vi "client-test2.vi"() -> ()   [LabVIEW 2016]
doc: "client test for TCP server in Main."
uses:
  <vilib>/NI/STM/TCP/TCP Read Options.ctl
  <vilib>/NI/STM/TCP/Read Meta Data (TCP Ref).vi
  <vilib>/NI/STM/TCP/Get Connection Reference (TCP).vi
  <vilib>/NI/STM/TCP/Read Meta Data (TCP Clst).vi
  <vilib>/NI/STM/TCP/Read Message (TCP).vi
  <vilib>/NI/STM/NI STM.lvlib
  <vilib>/NI/STM/TCP/Write Message (TCP).vi
panel:
  out "data string":string
  out "error  out":errorcluster
  in  "stop":bool
  in  "Target IP Address":string="localhost"
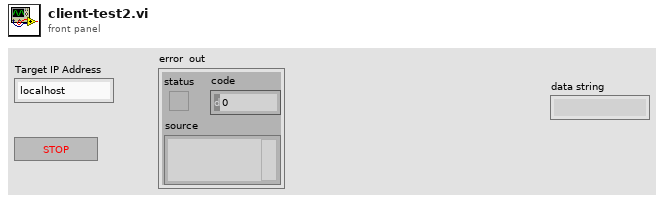
[diagram p1: front panel]
types:
  T1 = typedef "NI STM.lvlib/TCP Connection Info.ctl" = cluster{"connection ID":refnum<k5>, "meta data":T2[]}
  T2 = typedef "NI STM.lvlib/MetaDataElement.ctl" = string
  T3 = typedef "NI STM.lvlib/TCP Read Options.ctl" = cluster{"ignore timeout error":bool, "timeout ms (1000)":i32}
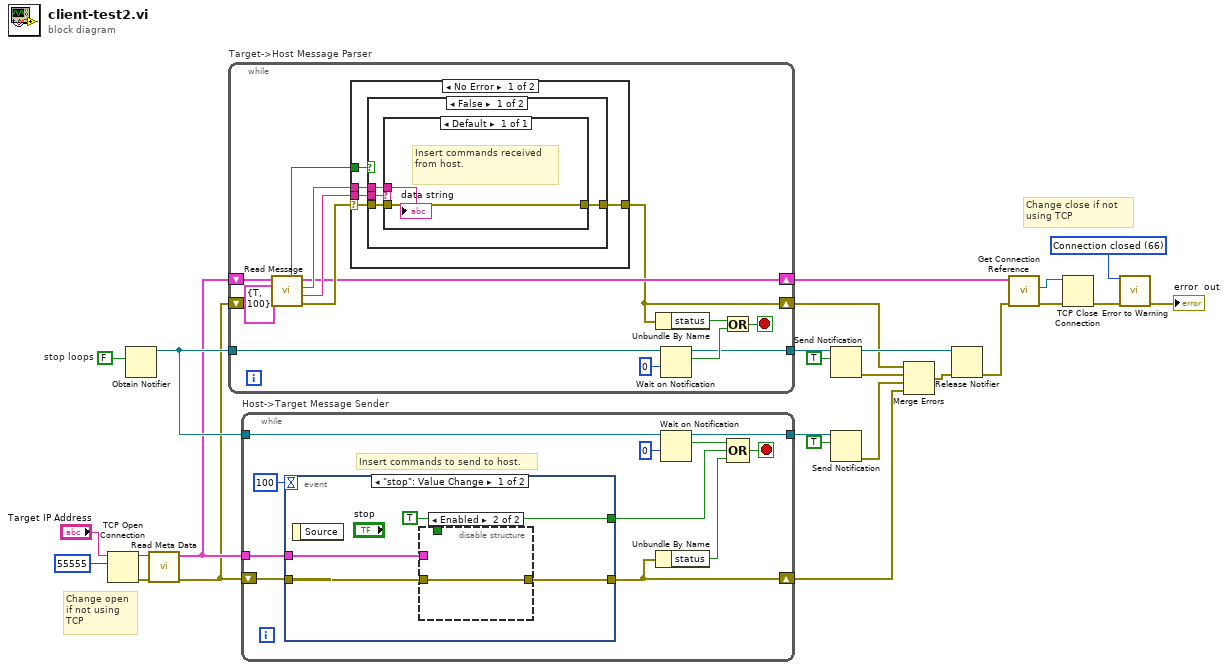
[diagram p0: block diagram]
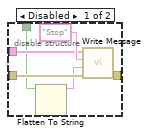
[diagram p2: hidden frame]
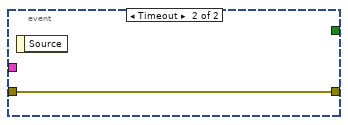
[diagram p3: hidden frame]
diagram:
  w11 = FALSE  # stop loops
  w23 = 66 items=["No Error", "Argument Error", "Memory Full", "Out of Zone", "End of File", "File Already Open", "Generic File IO Error", "File Not Found", "File Permission Error", "Disk Full", "Duplicate Path", "Too Many Files Open", "Not Enabled", "Resource File Not Found", "Cannot Add Resource", "Resource Not Found", "Image Not Found", "Image Memory Error", "Pen Does Not Exist", "Config Bad Type", "Config Token Not Found", "Config Parse Error", "Config Memory Error", "Bad External Code Format", "Bad External Code Offset", "External Code Not Present", "Null Window", "Destroy Window Mixup", "Null Menu", "Print Aborted", "Bad Print Record", "Print Driver Error", "Windows Error During Print", "Memory Error During Print", "Print Dialog Error", "Generic Print Error", "Invalid Device Refnum", "Device Not Found", "Device Parameter Error", "Device Unit Error", "Can't Open Device", "Device Call Aborted", "Generic Error", "Cancelled By User", "Object ID Too Low", "Object ID Too High", "Object Not In Heap", "Unknown Heap", "Bad DefProc ID", "DefProc Not In Table", "Message Out Of Range", "Null Method", "Unknown Message", "Manager Call Not Supported", "Bad address", "Connection In progress", "Connection timed out", "Connection is already in progress", "Network attribute not supported", "Network error", "Address in use", "System out of memory", "Connection aborted", "Connection refused", "Connection is not connected", "Connection is already connected", "Connection closed", "Initialize error (interapplication manager)", "Bad occurrence", "Wait on unbound occurrence handler", "Occurrence queue overflow", "Bad path", "Semaphore not signaled", "Unrecognized type (interapplication manager)"] ("1st Error to Convert")
  # "Change close if not using TCP"
  # "Change open if not using TCP"
  n1 = TCP Open Connection(address="Target IP Address", remote port or service name=u16 55555 ("remote port")) -> (connection ID=w7:refnum<k5>, error out=w6:errorcluster)  [unwired: 1 in, 2 out]
  n2 = Obtain Notifier(notification data type=w11) -> (notifier out=w14:refnum<notifier>)  [unwired: 3 in, 2 out]
  n3 = call-poly <vilib>:"Read Meta Data.vi"("error in"=w6, "connection ID"=w7) -> ("error out"=w8:errorcluster, "connection info out"=w9:T1)  [unwired: 1 in, 7 out]
  n4 = while "Target->Host Message Parser" {
    shift-right: [w27] -> w3
    shift-left: w8 -> [w39]
    tunnel: w14 -> [w33]
    tunnel: [w29] -> w12
    shift-right: [w34] -> w10
    shift-left: w9 -> [w40]
    stop <- w30 stop-if-true
    n5 = call-poly <vilib>:"Read Message.vi"("options"=T3 {"ignore timeout error"=TRUE, "timeout ms (1000)"=100}, "error in"=w39, "connection info in"=w40) -> ("error out"=w35:errorcluster, "name"=w38:T2, "data string"=w37:string, "connection info out"=w34:T1, "timed out?"=w36:bool)  [unwired: 2 in, 2 out]
    n6 = case shown="No Error" w35 {
      selector: w35 -> [w42 w53]
      tunnel: w38 -> [w45 _]
      tunnel: w37 -> [w44 _]
      tunnel: w36 -> [w43 _]
      tunnel: [w41 w53] -> w27
      frame No Error {
        n7 = case shown="False" w43 {
          tunnel: w45 -> [w46 _]
          tunnel: w44 -> [w49 _]
          tunnel: w42 -> [w48 w52]
          tunnel: [w47 w52] -> w41
          frame False {
            n8 = case shown="Default" w46 {
              tunnel: w49 -> [w50]
              tunnel: w48 -> [w51]
              tunnel: [w51] -> w47
              frame Default {
                # "Insert commands received from host."
                "data string" <- w50
              }
            }
          }
          frame True {
          }
        }
      }
      frame Error {
      }
    }
    n9 = Unbundle By Name(w27) -> ("status"=w28:bool)
    n10 = Wait on Notification(notifier=w33, timeout in ms (-1)=0) -> (notifier out=w29:refnum<notifier>, notification=w31:bool)  [unwired: 2 in, 2 out]
    n11 = Or(x=w28, y=w31) -> (x .or. y?=w30:bool)
  }
  n12 = while "Host->Target Message Sender" {
    shift-right: [w56] -> w17
    shift-left: w8 -> [w64]
    tunnel: w9 -> [w63]
    tunnel: w14 -> [w60]
    tunnel: [w57] -> w15
    stop <- w58 stop-if-true
    # "Insert commands to send to host."
    n13 = event shown="[0] \"stop\": Value Change" {
      selector: _ -> [_ _]
      dyn-events: _ -> [_ _]
      timeout: 100 -> [_ _]
      tunnel: w63 -> [w68 _]
      tunnel: w64 -> [w67 w76]
      tunnel: [w66 _] -> w55
      tunnel: [w65 w76] -> w56
      event "stop": Value Change {
        w66 = TRUE ("stop")
        n14 = event-data() -> ()  [unwired: 2 out]
        n15 = disable-structure shown="Enabled" {
          disable-tunnel: w68 -> [w73 _]
          disable-tunnel: w67 -> [w72 w75]
          disable-tunnel: w66 -> [w70 _]
          disable-tunnel: [w69 w75] -> w65
          frame Disabled {
            n16 = Flatten To String(anything=w70) -> (data string=w71:string)  [unwired: 2 in, 3 out]
            n17 = call-poly <vilib>:"Write Message.vi"("error in"=w72, "data"=w71, "name"="Stop" ("Name"), "connection info in"=w73) -> ("error out"=w69:errorcluster)  [unwired: 1 in, 6 out]
          }
          frame Enabled {
          }
        }
      }
      event Timeout {
        n18 = event-data() -> ()  [unwired: 2 out]
      }
    }
    n19 = Unbundle By Name(w56) -> ("status"=w54:bool)
    n20 = Wait on Notification(notifier=w60, timeout in ms (-1)=0) -> (notifier out=w57:refnum<notifier>, notification=w62:bool)  [unwired: 2 in, 2 out]
    n21 = Compound Arithmetic op=OR(w62, w55, w54) -> (w58:bool)
  }
  n22 = Send Notification(notification=TRUE, notifier=w12) -> (notifier out=w20:refnum<notifier>, error out=w19:errorcluster)  [unwired: 1 in]
  n23 = Send Notification(notification=TRUE, notifier=w15) -> (error out=w18:errorcluster)  [unwired: 1 in, 1 out]
  n24 = Merge Errors(w3, w19, w18, w17) -> (w21:errorcluster)
  n25 = Release Notifier(notifier=w20, error in (no error)=w21) -> (error out=w22:errorcluster)  [unwired: 1 in, 2 out]
  n26 = call-poly <vilib>:"Get Connection Reference.vi"("error in"=w22, "connection info in"=w10) -> ("error out"=w2:errorcluster, "connection ID out"=w1:refnum<k5>)  [unwired: 8 out]
  n27 = TCP Close Connection(connection ID=w1, error in (no error)=w2) -> (error out=w24:errorcluster)  [unwired: 2 out]
  n28 = call <vilib>:"Error to Warning.vi"("1st Error to Convert"=w23, "error in"=w24) -> ("warning out"=→"error  out":errorcluster)  [unwired: 3 in, 10 out]
